vi "Update from Variants.vi"(6 "Timestamp (Now)":dbl, 8 "error in (no error)":errorcluster, 10 "Variants":variant[](array[variant]), 11 "StringGroup in":refnum<class "StringGroup.lvclass">) -> (0 "error out":errorcluster, 3 "StringGroup out":refnum<class "StringGroup.lvclass">)   [LabVIEW 2020, in "Vecto.lvlib" / "StringGroup.lvclass"]
uses:
  StringGroup.lvclass
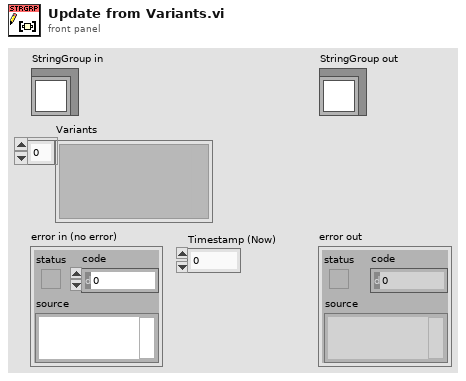
[diagram p1: front panel]
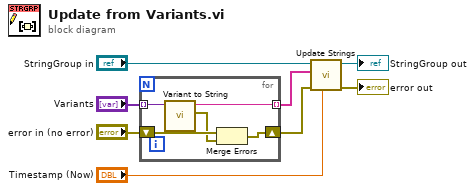
[diagram p0: block diagram]
diagram:
  n1 = for {
    tunnel: "Variants" -> [w13] mode=indexing
    shift-right: [w10] -> w4
    shift-left: "error in (no error)" -> [w12]
    tunnel: [w9] -> w5 mode=indexing
    n2 = call "Variant to String.vi"("Variant"=w13) -> ("error out"=w11:errorcluster, "String"=w9:string)  [unwired: 9 in]
    n3 = Merge Errors(w12, w11) -> (w10:errorcluster)
  }
  n4 = call "Update Strings.vi"("Timestamp (Now)"="Timestamp (Now)", "error in (no error)"=w4, "Strings"=w5, "StringGroup in"="StringGroup in") -> ("error out"=→"error out":errorcluster, "StringGroup out"=→"StringGroup out":refnum<class "StringGroup.lvclass">)  [unwired: 6 in]
